vi "Populate Device Names.vi"(8 "error in (no error)":errorcluster, 11 "RESOURCE NAME Ref":refnum<vi>) -> (0 "error out":errorcluster, 3 "RESOURCE NAME Ref out":refnum<vi>)   [LabVIEW 2025, in "I2C Bus Monitor UI.lvlib"]
uses:
  I2C Bus Monitor UI.lvlib
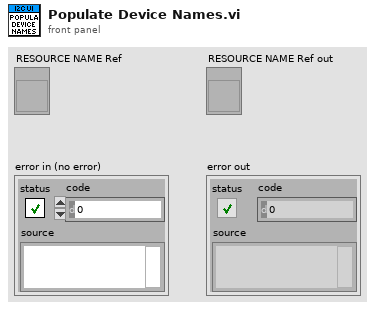
[diagram p1: front panel]
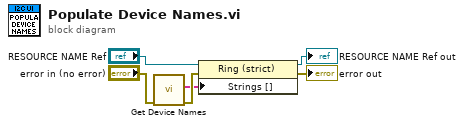
[diagram p0: block diagram]
diagram:
  n1 = call "Get Device Names.vi"("error in (no error)"="error in (no error)") -> ("error out"=w6:errorcluster, "Alias"=w4:string[])  [unwired: 8 in, 1 out]
  n2 = property on="Property Node" class="Ring (strict)"(reference="RESOURCE NAME Ref", error in=w6, "Strings []"=w4) -> (reference out=→"RESOURCE NAME Ref out":refnum<vi>, error out=→"error out":errorcluster)
